vi "outPutTestCaseArrayInCanFile.vi"(8 "error in":errorcluster, 11 "tbl":string[][](table)) -> (0 "error out":errorcluster, 3 "testCaseInCanFileArr":string[](array[string]))   [LabVIEW 2010]
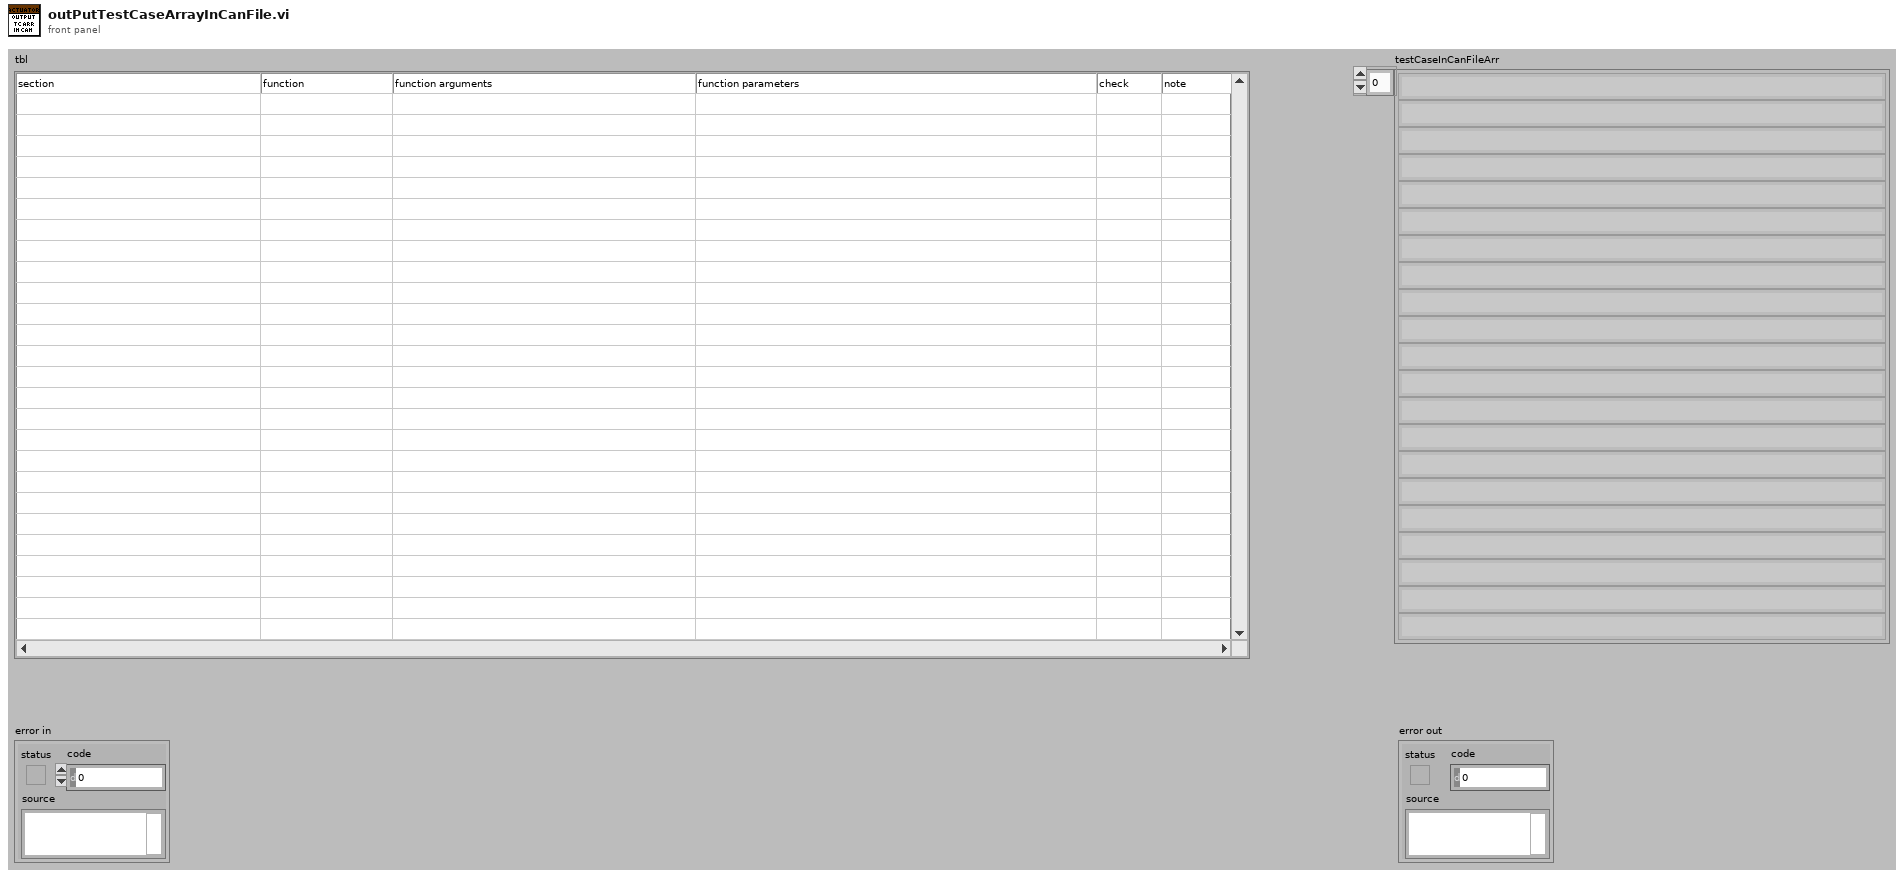
[diagram p1: front panel]
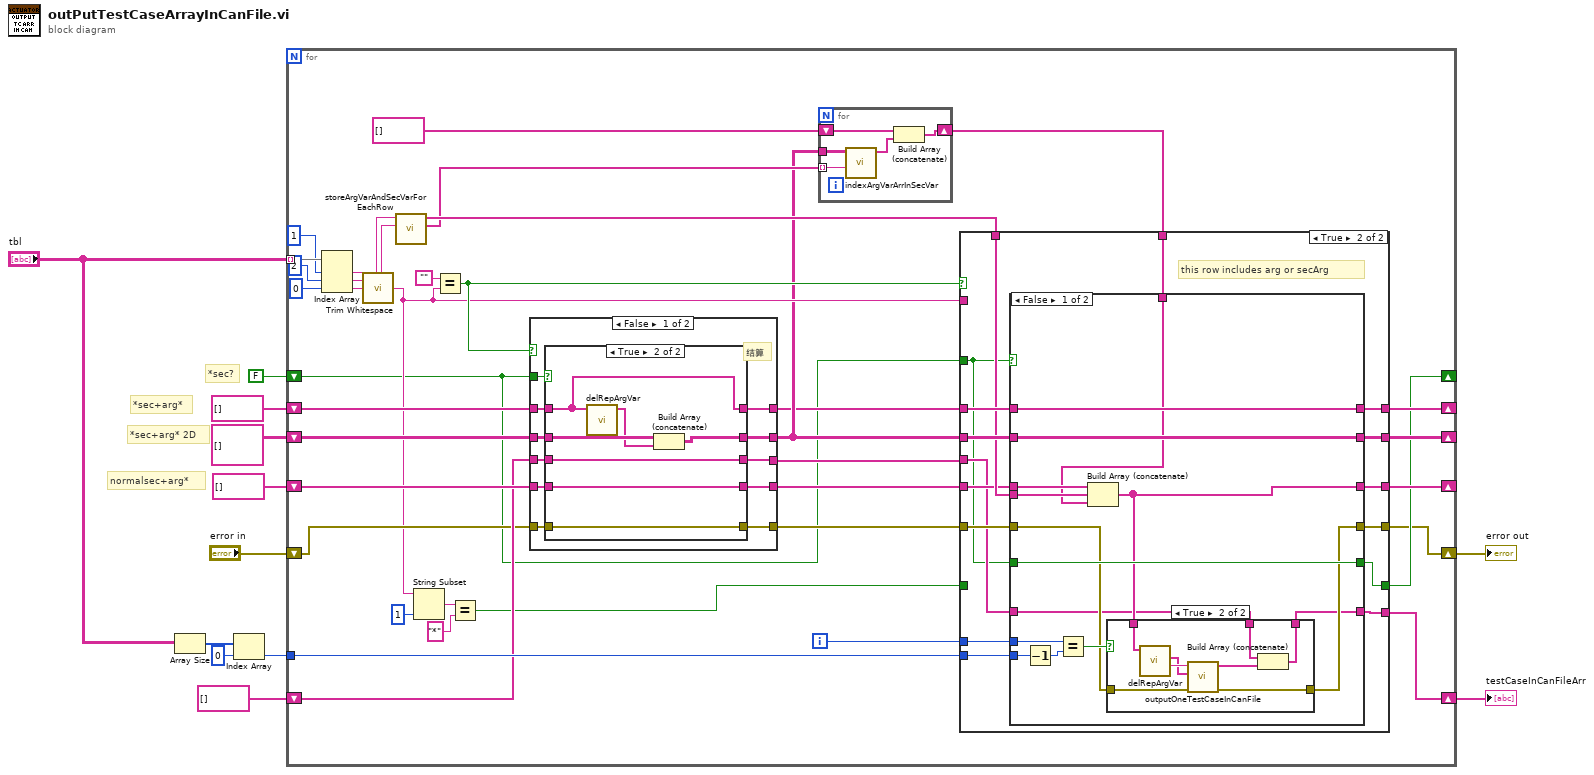
[diagram p0: block diagram]
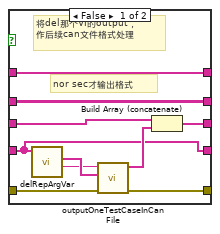
[diagram p2: hidden frame]
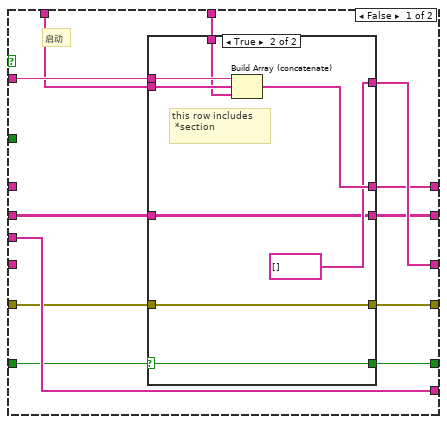
[diagram p4: hidden frame]
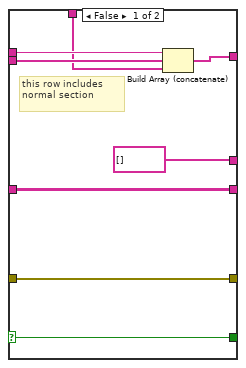
[diagram p5: hidden frame]
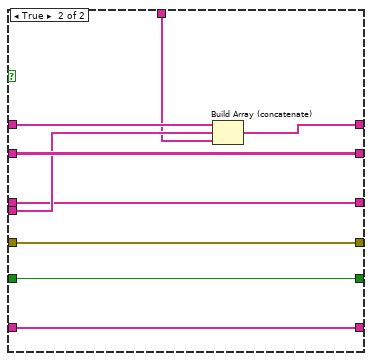
[diagram p7: hidden frame]
diagram:
  # "*sec?"
  # "*sec+arg* 2D"
  # "*sec+arg*"
  # "normalsec+arg*"
  n1 = Array Size(array="tbl") -> (size(s)=w3:i32[])
  n2 = Index Array(array=w3, index=0) -> (element=w1:i32)
  n3 = for {
    tunnel: "tbl" -> [w49] mode=indexing
    shift-right: [w40] -> _
    shift-left: string[] [] -> [w26]
    shift-right: [w35] -> _
    shift-left: string[] [] -> [w22]
    shift-right: [w36] -> _
    shift-left: string[][] [] -> [w24]
    shift-right: [w34] -> _
    shift-left: FALSE ("x = y?") -> [w13]
    shift-right: [w32] -> w5
    shift-left: "error in" -> [w23]
    shift-right: [w31] -> w6
    shift-left: string[] [] -> [w25]
    tunnel: w1 -> [w30]
    i -> [w29]
    n4 = Index Array(array=w49, index #1=1 ("index"), index #2=2 ("index"), index #3=0 ("index")) -> (element #1=w42:string, element #2=w43:string, element #3=w46:string)
    n5 = call <vilib>:"Trim Whitespace.vi"("string"=w46) -> ("trimmed string"=w19:string)  [unwired: 1 in]
    n6 = call "storeArgVarAndSecVarForEachRow.vi"("allArguments"=w43, "func"=w42) -> ("secVar"=w27:string[], "argVar"=w41:string[])  [unwired: 8 in]
    n7 = String Subset(string=w19, length (rest)=1 ("length (rest)")) -> (substring=w38:string)  [unwired: 1 in]
    n8 = Equal?(x="", y=w19) -> (x = y?=w20:bool)
    n9 = Equal?(x=w38, y="*") -> (x = y?=w17:bool)
    n10 = case shown="False" w20 {
      tunnel: w26 -> [w60 w79]
      tunnel: w25 -> [w59 w82]
      tunnel: w24 -> [w58 w81]
      tunnel: w23 -> [w57 w78]
      tunnel: w22 -> [w56 w80]
      tunnel: w13 -> [w55 _]
      tunnel: [w54 w82] -> w16
      tunnel: [w53 w81] -> w18
      tunnel: [w52 w78] -> w21
      tunnel: [w51 w80] -> w15
      tunnel: [w50 w79] -> w14
      frame False {
        # "结算"
        n11 = case shown="True" w55 {
          tunnel: w60 -> [w61 w71]
          tunnel: w56 -> [w62 w72]
          tunnel: w58 -> [w70 w77]
          tunnel: [w70 w75] -> w53
          tunnel: w57 -> [w67 w74]
          tunnel: [w66 w74] -> w52
          tunnel: w59 -> [w65 w73]
          tunnel: [w63 w73] -> w54
          tunnel: [w62 w72] -> w51
          tunnel: [w61 w71] -> w50
          frame False {
            # "nor sec才输出格式"
            # "将del那个VI的output，\n作后续can文件格式处理"
            n12 = call "delRepArgVar.vi"("sec+*var"=w61) -> ("sec"=w68:string, "*varNoRepeatArr"=w69:string[])  [unwired: 8 in, 1 out]
            n13 = call "outputOneTestCaseInCanFile.vi"("error in"=w67, "*varNoRepeatArr"=w69, "secName"=w68) -> ("error out"=w66:errorcluster, "oneTestCaseInCanFile"=w64:string[])  [unwired: 7 in]
            n14 = Build Array (concatenate)(w65, w64) -> (w63:string[])
          }
          frame True {
            n15 = call "delRepArgVar.vi"("sec+*var"=w72) -> ("sec+*varNoRepeatArr"=w76:string[])  [unwired: 8 in, 2 out]
            n16 = Build Array (concatenate)(w77, w76) -> (w75:string[][])
          }
        }
      }
      frame True {
        # "不结算"
      }
    }
    n17 = for {
      tunnel: w27 -> [w87] mode=indexing
      tunnel: w18 -> [w86]
      shift-right: [w83] -> w28
      shift-left: string[] [] -> [w85]
      n18 = call "indexArgVarArrInSecVar.vi"("*sec"=w87, "*sec+arg* 2D"=w86) -> ("argVarArrIn*sec"=w84:string[])  [unwired: 9 in]
      n19 = Build Array (concatenate)(w85, w84) -> (w83:string[])
    }
    n20 = case shown="True" w20 {
      tunnel: w19 -> [w98 _]
      tunnel: w14 -> [_ w126]
      tunnel: [w99 w125] -> w40
      tunnel: w41 -> [w97 w128]
      tunnel: w15 -> [_ w129]
      tunnel: w18 -> [w89 w130]
      tunnel: [w96 w131] -> w36
      tunnel: [w95 w127] -> w35
      tunnel: [w94 w119] -> w34
      tunnel: w13 -> [_ w120]
      tunnel: w28 -> [w93 w116]
      tunnel: w21 -> [w90 w124]
      tunnel: [w92 w123] -> w32
      tunnel: w16 -> [w91 w122]
      tunnel: [w91 w121] -> w31
      tunnel: w30 -> [_ w118]
      tunnel: w29 -> [_ w117]
      tunnel: w17 -> [w88 _]
      frame False {
        # "启动"
        n21 = case shown="True" w88 {
          selector: w88 -> [w104 w112]
          tunnel: [w105 string[] []] -> w99
          tunnel: w98 -> [w107 w115]
          tunnel: w97 -> [w106 w114]
          tunnel: [w102 w109] -> w96
          tunnel: [string[] [] w113] -> w95
          tunnel: [w104 w112] -> w94
          tunnel: w93 -> [w103 w111]
          tunnel: w89 -> [w102 w109]
          tunnel: w90 -> [w100 w108]
          tunnel: [w100 w108] -> w92
          frame False {
            # "this row includes \nnormal section"
            n22 = Build Array (concatenate)(w107, w106, w103) -> (w105:string[])
          }
          frame True {
            # "this row includes\n *section"
            n23 = Build Array (concatenate)(w115, w114, w111) -> (w113:string[])
          }
        }
      }
      frame True {
        # "this row includes arg or secArg"
        n24 = case shown="False" w120 {
          tunnel: [w144 w165] -> w131
          tunnel: w130 -> [w144 w165]
          tunnel: w129 -> [w143 w164]
          tunnel: w128 -> [w145 w163]
          tunnel: [w143 w162] -> w127
          tunnel: w126 -> [w146 w161]
          tunnel: [w135 w161] -> w125
          tunnel: w124 -> [w137 w160]
          tunnel: [w136 w160] -> w123
          tunnel: w122 -> [w134 w159]
          tunnel: [w133 w159] -> w121
          tunnel: w120 -> [w142 w158]
          tunnel: [w142 w158] -> w119
          tunnel: w118 -> [w140 _]
          tunnel: w117 -> [w141 _]
          tunnel: w116 -> [w132 w157]
          frame False {
            n25 = Decrement(x=w140) -> (x-1=w139:i32)
            n26 = Equal?(x=w141, y=w139) -> (x = y?=w138:bool)
            n27 = Build Array (concatenate)(w146, w145, w132) -> (w135:string[])
            n28 = case shown="True" w138 {
              tunnel: w135 -> [_ w156]
              tunnel: w137 -> [w148 w153]
              tunnel: [w148 w152] -> w136
              tunnel: w134 -> [w147 w151]
              tunnel: [w147 w149] -> w133
              frame False {
              }
              frame True {
                n29 = call "delRepArgVar.vi"("sec+*var"=w156) -> ("sec"=w155:string, "*varNoRepeatArr"=w154:string[])  [unwired: 8 in, 1 out]
                n30 = call "outputOneTestCaseInCanFile.vi"("error in"=w153, "*varNoRepeatArr"=w154, "secName"=w155) -> ("error out"=w152:errorcluster, "oneTestCaseInCanFile"=w150:string[])  [unwired: 7 in]
                n31 = Build Array (concatenate)(w151, w150) -> (w149:string[])
              }
            }
          }
          frame True {
            n32 = Build Array (concatenate)(w164, w163, w157) -> (w162:string[])
          }
        }
      }
    }
  }
  "testCaseInCanFileArr" <- w6
  "error out" <- w5
